vi "existDeviceByeBye.vi"(10 "USN":string, 11 "Item Names":string[](array[string])) -> (2 "index":i32, 3 "exist?":bool)   [LabVIEW 2010]
uses:
  <vilib>/regexp/Match Regular Expression.xnode
panel:
  in  "address":u32
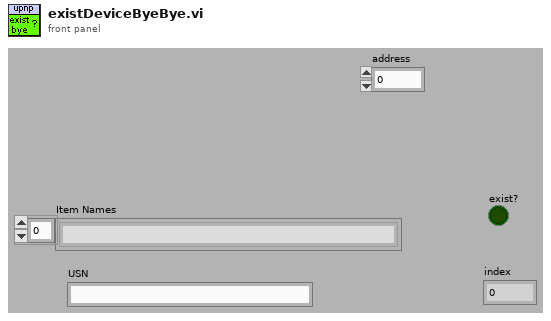
[diagram p1: front panel]
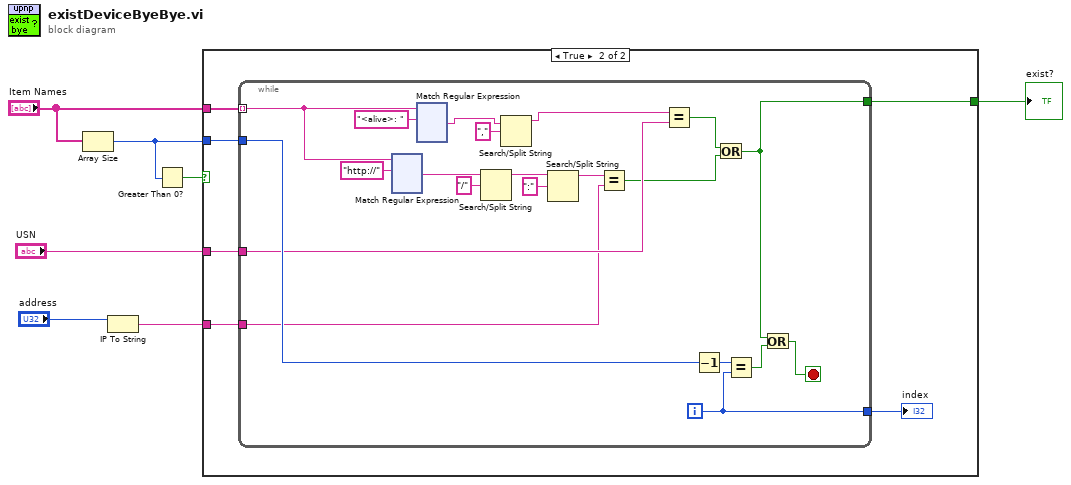
[diagram p0: block diagram]
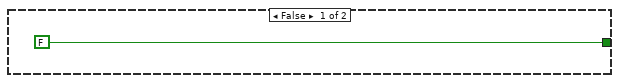
[diagram p2: hidden frame]
diagram:
  n1 = Array Size(array="Item Names") -> (size(s)=w6:i32)
  n2 = IP To String(2:"address") -> (0:w1:string)  [unwired: 1 out]
  n3 = Greater Than 0?(x=w6) -> (x > 0?=w4:bool)
  n4 = case shown="True" w4 {
    tunnel: "Item Names" -> [_ w14]
    tunnel: w6 -> [_ w13]
    tunnel: [FALSE w12] -> w5
    tunnel: "USN" -> [_ w11]
    tunnel: w1 -> [_ w9]
    frame False {
    }
    frame True {
      n5 = while {
        tunnel: w14 -> [w22] mode=indexing
        tunnel: [w15] -> w12
        tunnel: w13 -> [w32]
        tunnel: w11 -> [w31]
        tunnel: [w30] -> w10
        tunnel: w9 -> [w23]
        i -> [w30]
        stop <- w35 stop-if-true
        n6 = xnode "Match Regular Expression"("input string"=w22, "regular expression"="http://") -> ("after match"=w28:string)  [unwired: 2 in, 6 out]
        n7 = xnode "Match Regular Expression"("input string"=w22, "regular expression"="<alive>: ") -> ("after match"=w19:string)  [unwired: 2 in, 6 out]
        n8 = Search/Split String(string=w28, search string/char (-)="/") -> (substring before match=w26:string)  [unwired: 3 out]
        n9 = Search/Split String(string=w19, search string/char (-)=",") -> (substring before match=w18:string)  [unwired: 3 out]
        n10 = Search/Split String(string=w26, search string/char (-)=":") -> (substring before match=w24:string)  [unwired: 3 out]
        n11 = Equal?(x=w24, y=w23) -> (x = y?=w16:bool)
        n12 = Equal?(x=w18, y=w31) -> (x = y?=w17:bool)
        n13 = Decrement(x=w32) -> (x-1=w34:i32)
        n14 = Or(x=w17, y=w16) -> (x .or. y?=w15:bool)
        n15 = Equal?(x=w34, y=w30) -> (x = y?=w33:bool)
        n16 = Or(x=w15, y=w33) -> (x .or. y?=w35:bool)
      }
      "index" <- w10
    }
  }
  "exist?" <- w5
